vi "读取存储数据.vi"(8 "error in (no error)":errorcluster caption="错误输入（无错误）", 11 "数据存储输入":refnum<class "数据存储.lvclass">) -> (0 "error out":errorcluster caption="错误输出", 2 "采集数据":dbl[](array[numeric]), 3 "数据存储输出":refnum<class "数据存储.lvclass">)   [LabVIEW 2013, in "数据存储.lvclass"]
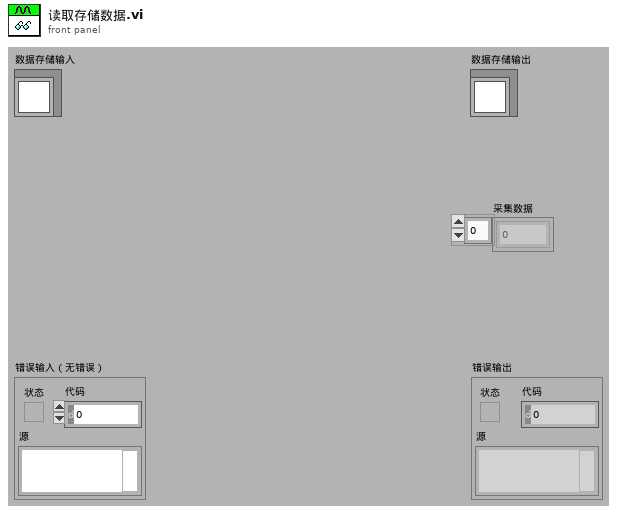
[diagram p1: front panel]
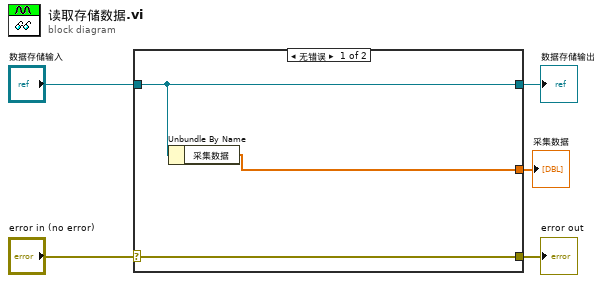
[diagram p0: block diagram]
diagram:
  n1 = case shown="无错误" "error in (no error)" {
    selector: "error in (no error)" -> [w8 w9]
    tunnel: [w8 w9] -> w4
    tunnel: [w7 w10] -> w2
    tunnel: "数据存储输入" -> [w7 w10]
    tunnel: [w6 _] -> w1
    frame No Error {
      n2 = Unbundle By Name(w7) -> ("采集数据"=w6:dbl[])
    }
    frame Error {
    }
  }
  "error out" <- w4
  "数据存储输出" <- w2
  "采集数据" <- w1
